vi "Change Include Seconds.vi"(8 "error in (no error)":errorcluster, 10 "Include Seconds?":bool, 11 "Numeric Data Type in":refnum<class "Numeric Data Type.lvclass">) -> (0 "error out":errorcluster, 3 "Numeric Data Type out":refnum<class "Numeric Data Type.lvclass">)   [LabVIEW 2018, in "Numeric Data Type.lvclass"]
uses:
  Numeric Data Type.lvclass
  Numeric Data Type.lvclass/Numeric Data Type.ctl
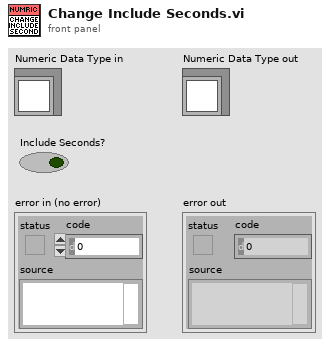
[diagram p1: front panel]
types:
  T1 = typedef "Numeric Data Type.lvclass/Time Info.ctl" = cluster{"Time Format":T2, "Numeric Format":T3, "Clock Type":T4, "Include Seconds?":bool, "Seconds Precision":i16, "Date Order":T5, "Date Format":T6, "Year Format":T7, "UTC":i16}
  T2 = typedef "Numeric Data Type.lvclass/Time Format.ctl" = enum16{"Custom time format", "System time format", "Time unused"}
  T3 = typedef "Numeric Data Type.lvclass/Numeric Format Enum.ctl" = enum16{"Floating Point Notation", "Scientific Notation", "Engineering Notation", "SI Notation", "<not used>", "Decimal", "Hexadecimal", "Octal", "Binary", "<not used 2>", "Absolute Time", "Relative Time"}
  T4 = typedef "Numeric Data Type.lvclass/Clock Type.ctl" = enum32{"12-Hour (AM/PM)", "24-Hour"}
  T5 = typedef "Numeric Data Type.lvclass/Date Order.ctl" = enum32{"M/D/Y", "D/M/Y", "Y/M/D"}
  T6 = typedef "Numeric Data Type.lvclass/Date Format.ctl" = enum16{"Custom date format", "System date format", "Date unused"}
  T7 = typedef "Numeric Data Type.lvclass/Year Format.ctl" = enum32{"No Year", "2-digit Year", "4-digit Year"}
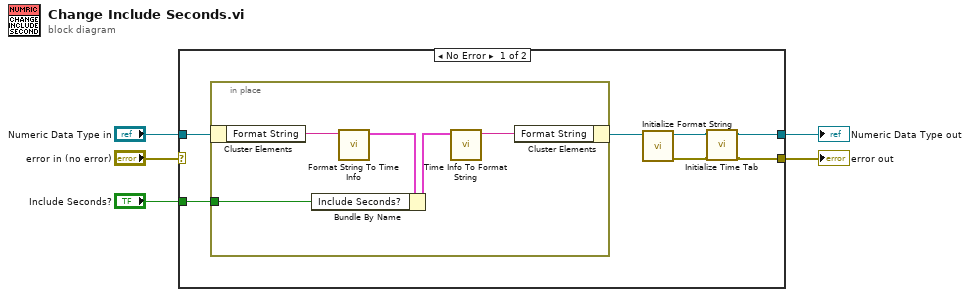
[diagram p0: block diagram]
diagram:
  n1 = case shown="No Error" "error in (no error)" {
    selector: "error in (no error)" -> [_ w19]
    tunnel: [w7 w19] -> w4
    tunnel: [w9 w18] -> w2
    tunnel: "Numeric Data Type in" -> [w12 w18]
    tunnel: "Include Seconds?" -> [w6 _]
    frame No Error {
      n2 = in-place {
        in-place-border: w6 -> [w13]
        n3 = in-place-cluster #1(w12) -> ("Format String"=w17:string)
        n4 = call "Format String To Time Info.vi"("Format String"=w17) -> ("Time Info"=w16:T1)  [unwired: 10 in]
        n5 = Bundle By Name(cluster=w16, "Include Seconds?"=w13) -> (w15:T1)
        n6 = call "Time Info To Format String.vi"("Time Format & Precision Info"=w15) -> ("Format String"=w14:string)  [unwired: 10 in]
        n7 = in-place-cluster #1("Format String"=w14) -> (w11:refnum<class "Numeric Data Type.lvclass">)
      }
      n8 = call "Initialize Format String.vi"("Numeric Data Type in"=w11) -> ("error out"=w8:errorcluster, "Numeric Data Type (dup)"=w10:refnum<class "Numeric Data Type.lvclass">)  [unwired: 9 in]
      n9 = call "Initialize Time Tab.vi"("error in (no error)"=w8, "Numeric Data Type in"=w10) -> ("error out"=w7:errorcluster, "Numeric Data Type (dub)"=w9:refnum<class "Numeric Data Type.lvclass">)  [unwired: 8 in]
    }
    frame Error {
    }
  }
  "error out" <- w4
  "Numeric Data Type out" <- w2
